vi "DHE_LoadImgparams.vi"(8 "error in (no error)":errorcluster) -> (0 "error out":errorcluster, 1 "basename":string="LASTIMG", 2 "dir":string="LASTIMG", 3 "froot":string="LASTIMG", 4 "number":i32, 5 "sufix":string="LASTIMG", 7 "prefix":string="LASTIMG")   [LabVIEW 2016]
uses:
  <vilib>/Utility/config.llb/Read Key (String).vi
  <vilib>/Utility/config.llb/Read Key (I32).vi
  <vilib>/Utility/config.llb/NI_LVConfig.lvlib
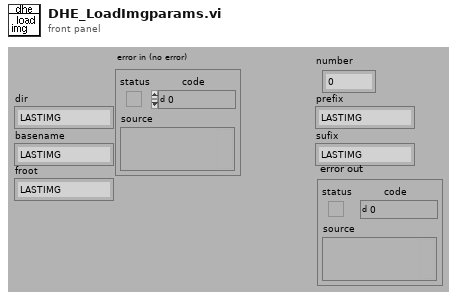
[diagram p1: front panel]
types:
  T1 = typedef "NI_LVConfig.lvlib/Config Data RefNum.ctl" = refnum<k1>
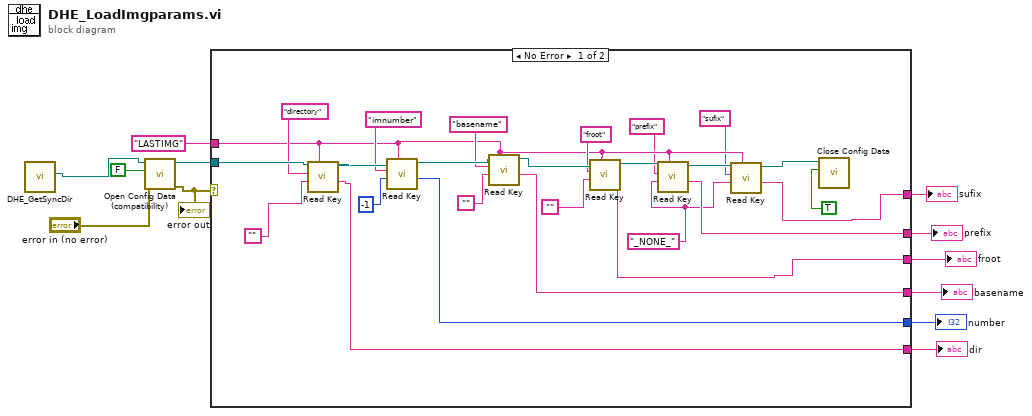
[diagram p0: block diagram]
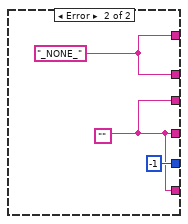
[diagram p2: hidden frame]
diagram:
  n1 = call "DHE_GetSyncDir.vi"() -> ("sync file"=w1:path)  [unwired: 11 out]
  n2 = call <vilib>:"Open Config Data (compatibility).vi"("error in (no error)"="error in (no error)", "create file if necessary (T)"=FALSE ("create file if necessary? (T)"), "configuration file path"=w1) -> ("error out"=w9:errorcluster, "refnum"=w12:T1)  [unwired: 6 in, 1 out]
  "error out" <- w9
  n3 = case shown="No Error" w9 {
    tunnel: w12 -> [w38 _]
    tunnel: "LASTIMG" ("section") -> [w19 _]
    tunnel: [w32 w40] -> w8
    tunnel: [w29 -1 ("value")] -> w7
    tunnel: [w26 w40] -> w6
    tunnel: [w24 w40] -> w5
    tunnel: [w15 w39] -> w4
    tunnel: [w14 w39] -> w3
    frame No Error {
      w13 = "_NONE_" ("sufix")
      n4 = call-poly <vilib>:"Read Key.vi"("section"=w19, "default value"="", "key"="directory", "refnum"=w38) -> ("value"=w32:string, "refnum out"=w37:T1)  [unwired: 2 in, 4 out]
      n5 = call-poly <vilib>:"Read Key.vi"("section"=w19, "default value"=-1 ("number"), "key"="imnumber", "refnum"=w37) -> ("value"=w29:i32, "refnum out"=w35:T1)  [unwired: 1 in, 5 out]
      n6 = call-poly <vilib>:"Read Key.vi"("section"=w19, "default value"="", "key"="basename", "refnum"=w35) -> ("value"=w26:string, "refnum out"=w34:T1)  [unwired: 2 in, 4 out]
      n7 = call-poly <vilib>:"Read Key.vi"("section"=w19, "default value"="", "key"="froot", "refnum"=w34) -> ("value"=w24:string, "refnum out"=w22:T1)  [unwired: 2 in, 4 out]
      n8 = call-poly <vilib>:"Read Key.vi"("section"=w19, "default value"=w13, "key"="prefix", "refnum"=w22) -> ("value"=w15:string, "refnum out"=w21:T1)  [unwired: 2 in, 4 out]
      n9 = call-poly <vilib>:"Read Key.vi"("section"=w19, "default value"=w13, "key"="sufix", "refnum"=w21) -> ("value"=w14:string, "refnum out"=w20:T1)  [unwired: 2 in, 4 out]
      n10 = call <vilib>:"Close Config Data.vi"("write file if changed (T)"=TRUE ("write configuration file? (F)"), "refnum"=w20) -> ()  [unwired: 1 in, 9 out]
    }
    frame Error {
      w39 = "_NONE_" ("sufix")
      w40 = ""
    }
  }
  "dir" <- w8
  "number" <- w7
  "basename" <- w6
  "froot" <- w5
  "prefix" <- w4
  "sufix" <- w3
